vi "Step 3 - Analyze Quantized Decimation (MRate).vi"() -> ()   [LabVIEW 2023]
doc: "Demonstrates how to use the DFD MRate FXP Quantization VI to quantize a floating-point decimation filter and how to use the DFD Plot MRate Freq Response VI to analyze the characteristics of the quantized filter."
uses:
  <vilib>/addons/Digital Filter Design/_Objects.llb/DFD Coef Norm Type.ctl
  <vilib>/addons/Digital Filter Design/NI_DigFilterLicensed.lvlib
panel:
  out "Magnitude Response":cluster{"f0":dbl, "df":dbl, "values":dbl[]}[](graph)
  # "Select Help>>Show Context Help and move the cursor over the VI icon for more information."
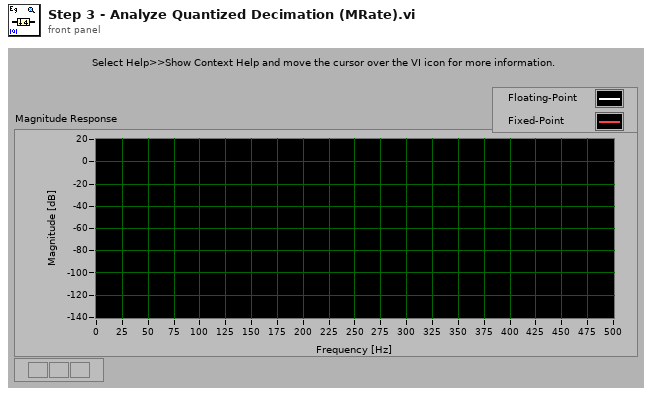
[diagram p1: front panel]
types:
  T1 = typedef "NI_DigFilterLicensed.lvlib/DFD Coef Norm Type.ctl" = enum16{"No Norm", "Time Domain 1-Norm", "Time Domain 2-Norm", "Time Domain Inf-Norm"}
  T2 = typedef "NI_DigFilterLicensed.lvlib/DFD Multirate Filter Obj.ctl" = cluster{"mMRate_Structure":enum16{"CIC", "FIR", "IIR", "Lattice"}, "mMRate_Mode":T3, "mMRate_Factor":i32, "mMRate_FIRParams":cluster{"mMRate_FIR_H":dbl[], "mMRate_FIR_IsNyquist?":bool, "mMRate_FIR_IsSymmetric?":bool}, "mMRate_CICParams":cluster{"mMRate_CIC_#Stage":i32, "mMRate_CIC_Lag":i32, "mMRate_CIC_Type":enum16{"Lowpass", "Highpass"}}, "mMRate_Order":i32, "mMRate_Version":string, "mMRate_Comments":string, "mMRate_RationalFactor":cluster{"mMRate_L":i32, "mMRate_M":i32}, "mMRate_Fs":dbl, "mMRate_Quantized?":bool, "mMRate_QFilterGain":dbl, "mMRate_CoefWl":i16, "mMRate_Scaling":cluster{"mMRate_ScaleByPowerOf2?":bool, "mMRate_ScaleType":T1}, "mMRate_InputWl":i16, "mMRate_OutputWl":i16, "mMRate_OutputMode":T4, "mMRate_MultMode":T5, "mMRate_BitPruning":bool, "mMRate_GainWl":i16, "mMRate_OutputFwl":i16, "mMRate_SumIwl":i16, "mMRate_InputIwl ":i16, "mMRate_SumWl":i16, "mMRate_CoefIwl":i16}
  T3 = typedef "NI_DigFilterLicensed.lvlib/DFD Multirate Mode.ctl" = i16
  T4 = typedef "NI_DigFilterLicensed.lvlib/DFD Round-off Mode.ctl" = enum16{"Nearest", "Truncation"}
  T5 = typedef "NI_DigFilterLicensed.lvlib/DFD FXP MRate Multiply Mode.ctl" = enum16{"Truncated", "Full"}
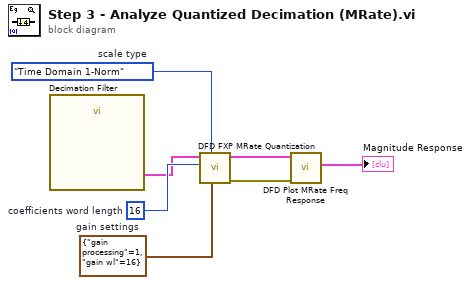
[diagram p0: block diagram]
diagram:
  w2 = i16 16  # coefficients word length
  w3 = cluster{"gain processing":u16, "gain wl":i16} {"gain processing"=1, "gain wl"=16}  # gain settings
  w7 = DFD_Coef_Norm_Type."Time Domain 1-Norm"  # scale type
  n1 = call "Decimation Filter"() -> ("multirate filter out"=w1:T2)  [unwired: 11 out]
  n2 = call <vilib>:"DFD FXP MRate Quantization.vi"("gain settings"=w3, "scale type"=w7, "coefficients word length"=w2, "multirate filter in"=w1) -> ("error out"=w5:errorcluster, "multirate filter out"=w6:T2)  [unwired: 2 in, 4 out]
  n3 = call <vilib>:"DFD Plot MRate Freq Response.vi"("error in (no error)"=w5, "multirate filter in"=w6) -> ("magnitude response"=→"Magnitude Response":cluster{"f0":dbl, "df":dbl, "values":dbl[]}[])  [unwired: 5 in, 4 out]
